vi "Run 5.vi"   [LabVIEW 2016]
types:
  T1 = typedef "LVHSConnector.ctl" = refnum<class "BrickReference.lvclass">
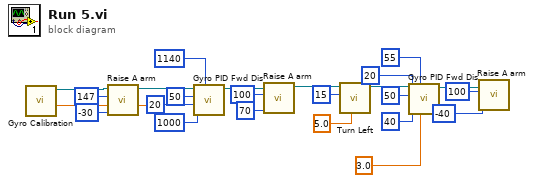
[diagram p0: block diagram]
diagram:
  n1 = call "Gyro Calibration.vi"() -> ("Degrees"=w16:sgl, "NXT/EV3"=w24:T1)  [unwired: 7 in, 1 out]
  n2 = call "Raise A arm.vi"("Power"=i8 -30, "Rotation"=147, "EV3 in"=w24) -> ("EV3 out"=w21:T1)  [unwired: 8 in]
  n3 = call "Gyro PID Fwd Dis.vi"("Target angle"=w16, "Threshold to stop"=1140, "Threshold to slow"=1000, "Min. speed"=20, "Max. speed"=50, "EV3 in"=w21) -> ("EV3 out"=w15:T1)  [unwired: 5 in]
  n4 = call "Raise A arm.vi"("Power"=i8 70, "Rotation"=100, "EV3 in"=w15) -> ("EV3 out"=w12:T1)  [unwired: 8 in]
  n5 = call "Turn Left.vi"("Turning angle"=sgl 5.0, "Motor B (right)"=i8 15, "EV3 in"=w12) -> ("EV3 out"=w9:T1)  [unwired: 8 in]
  n6 = call "Gyro PID Fwd Dis.vi"("Target angle"=sgl 3.0, "Threshold to stop"=55, "Threshold to slow"=40, "Min. speed"=20, "Max. speed"=50, "EV3 in"=w9) -> ("EV3 out"=w3:T1)  [unwired: 5 in]
  n7 = call "Raise A arm.vi"("Power"=i8 -40, "Rotation"=100, "EV3 in"=w3) -> ()  [unwired: 8 in, 1 out]
